vi "Get File Name.vi"(1 "Game Data":string="String") -> (0 "File Name":path)   [LabVIEW 2019]
uses:
  <vilib>/Rock Robotics/Network Tables/NT Read String.vi
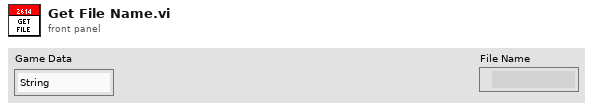
[diagram p1: front panel]
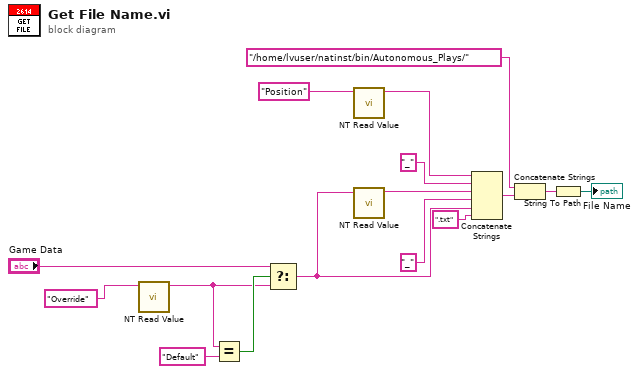
[diagram p0: block diagram]
diagram:
  n1 = call-poly <vilib>:"NT Read Value.vi"("Name"="Override") -> ("String"=w6:string)  [unwired: 9 in, 1 out]
  n2 = Equal?(x=w6, y="Default") -> (x = y?=w7:bool)
  n3 = Select(t="Game Data", s=w7, f=w6) -> (s? t:f=w1:string)
  n4 = call-poly <vilib>:"NT Read Value.vi"("Name"="Position") -> ("String"=w11:string)  [unwired: 9 in, 1 out]
  n5 = call-poly <vilib>:"NT Read Value.vi"("Name"=w1) -> ("String"=w4:string)  [unwired: 9 in, 1 out]
  n6 = Concatenate Strings(w11, "_" ("string"), w4, "_" ("string"), w1, ".txt" ("string")) -> (w13:string)
  n7 = Concatenate Strings("/home/lvuser/natinst/bin/Autonomous_Plays/" ("string"), w13) -> (w16:string)
  n8 = String To Path(string=w16) -> (path=→"File Name":path)
